vi "Scalar Bitpacked.vi"(8 "error in (no error)":errorcluster, 11 "Node Ptr":T1 format="%.0x") -> (0 "error out":errorcluster)   [LabVIEW 2015, in "FPGA Addon System Explorer.lvlib"]
uses:
  FPGA Addon System Explorer.lvlib
  <vilib>/NI Veristand/Custom Device API/Custom Device Item Ref.ctl
  Shared/FG Action.ctl
  <vilib>/NI Veristand/Custom Device API/Custom Device Channel.ctl
  <vilib>/NI Veristand/Custom Device API/Custom Device Channel Type.ctl
  Shared/Constants.vi
  <vilib>/NI Veristand/Custom Device API/Get Item Property (U32).vi
  <vilib>/NI Veristand/Custom Device API/NI VeriStand - Set Item Property.vi
  <vilib>/NI Veristand/Custom Device API/Set Item Property (U32).vi
  <vilib>/NI Veristand/Custom Device API/Get Item Property (String).vi
  <vilib>/NI Veristand/Custom Device API/Get Item Property (Variant).vi
  <vilib>/NI Veristand/Custom Device API/Set Item Property (Variant).vi
  <vilib>/NI Veristand/Custom Device Tools/Custom Device Utility Library/NI VeriStand - Search for All Items by GUID.vi
  <vilib>/NI VeriStand/Custom Device API/Custom Device API.lvlib
  Shared/FPGA Addon Shared.lvlib
  <vilib>/NI VeriStand/Custom Device Tools/Custom Device Utility Library/Custom Device Utility Library.lvlib
panel:
  out "Original Name":string
  in  "SHDocVw.IWebBrowser":refnum<k7>(container)
  in  "Reset":bool
  in  "Apply":bool
  in  "Number of Channels":u8
  in  "Header 2":cluster{"Section Name":string}={"Section Name"="Custom Device Item Settings"}
  in  "Header":cluster{"Section Name":string}={"Section Name"="Custom Device Item Settings"}
  in  "Description":string
  in  "Name":string
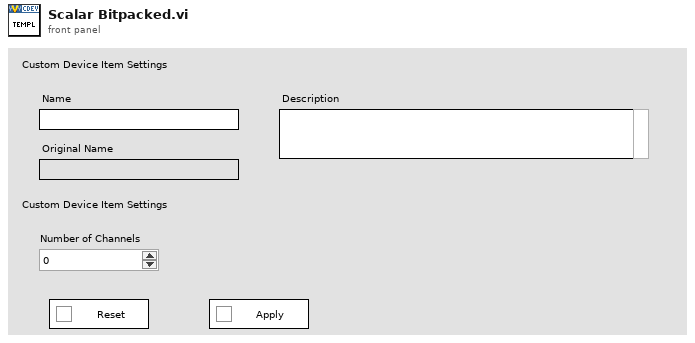
[diagram p1: front panel]
types:
  T1 = typedef "Custom Device API.lvlib/Custom Device Item Ref.ctl" = u64
  T2 = typedef "FPGA Addon Shared.lvlib/FG Action.ctl" = enum8{"GET", "SET"}
  T3 = typedef "FPGA Addon Shared.lvlib/Scalar Settings.ctl" = cluster{"Number of Channels":u8}
  T4 = typedef "FPGA Addon Shared.lvlib/Register Information.ctl" = cluster{"Name":string, "Data Type":T5, "Default Value":variant}
  T5 = typedef "FPGA Addon Shared.lvlib/Data Type.ctl" = enum8{"<Null>", "I8", "I16", "I32", "I64", "U8", "U16", "U32", "U64", "SGL", "Boolean", "Analog PWM In Settings", "Analog PWM In", "Digital PWM In Settings", "Digital PWM In", "Digital PWM Out", "Sine Out", "FXP+/-24.5", "FXP+/-16.5", "FXP+/-32.8", "FXP+/-64.32", "FXP+/-16.7", "FXP+/-20.5", "FXP+/-27.5", "FXP+/-32.16", "Digital Static In", "Digital Static Out", "Digital Static In Settings", "Digital WSS Out"}
  T6 = typedef "Custom Device API.lvlib/Custom Device Item Info.ctl" = cluster{"Name":string, "Is Channel":bool, "GUID":string, "Is Waveform":bool}
  T7 = typedef "Custom Device API.lvlib/Custom Device Channel.ctl" = cluster{"Type":T8, "Units":string, "Default Value":dbl, "Faultable":bool, "Scalable":bool}
  T8 = typedef "Custom Device API.lvlib/Custom Device Channel Type.ctl" = enum16{"Input", "Output"}
  T9 = typedef "Custom Device API.lvlib/Custom Device Commands.ctl" = enum16{"Default", "Item renamed", "Shutdown", "Dynamic button pressed"}
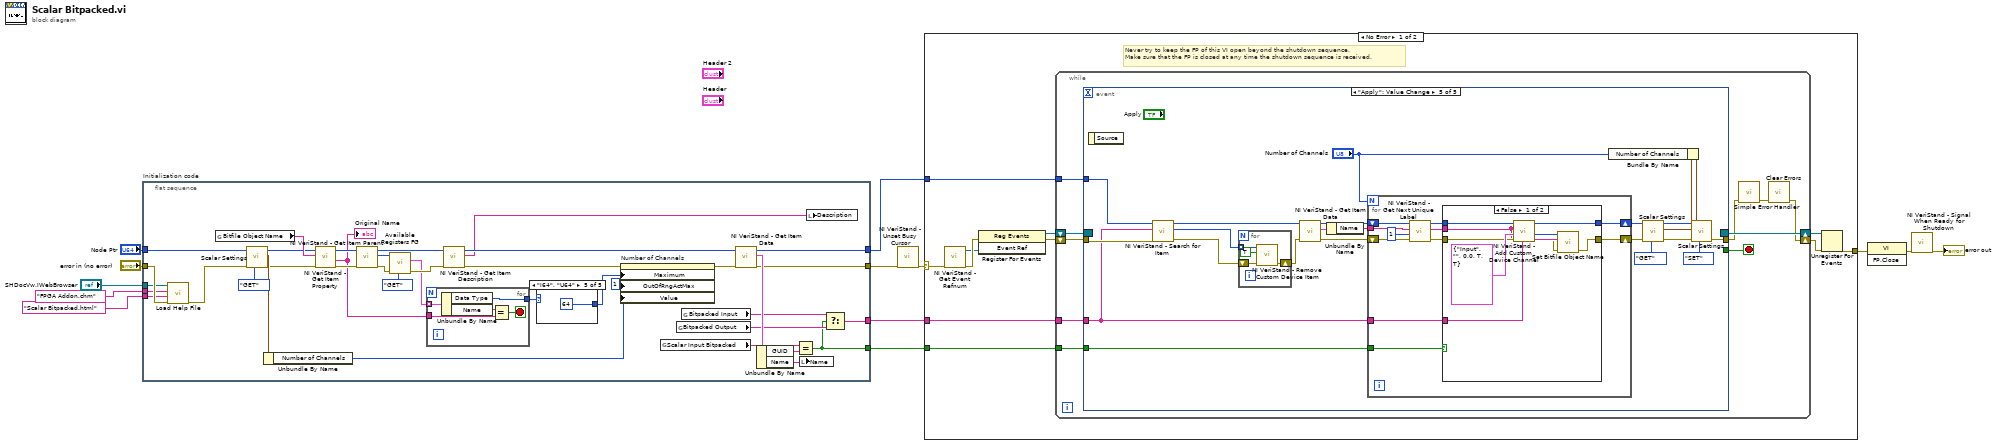
[diagram p0: block diagram]
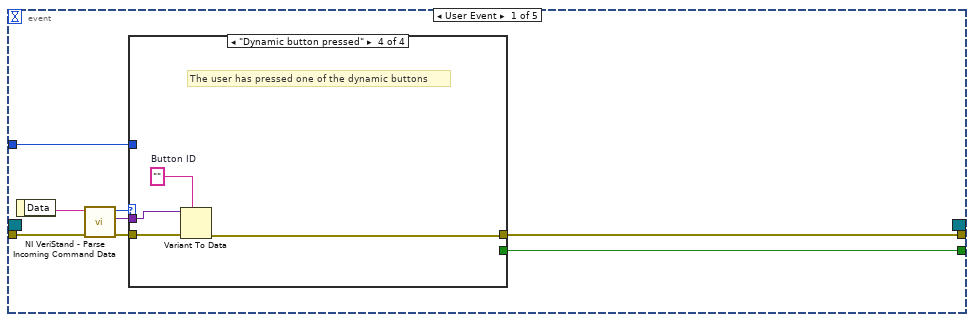
[diagram p2: hidden frame]
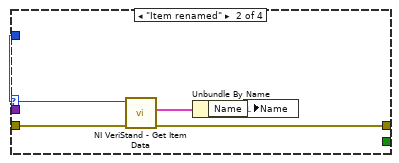
[diagram p4: hidden frame]
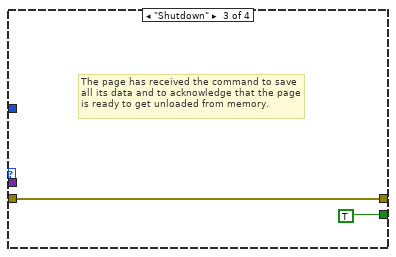
[diagram p5: hidden frame]
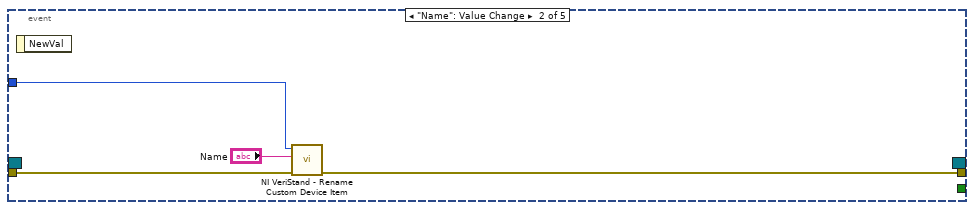
[diagram p6: hidden frame]
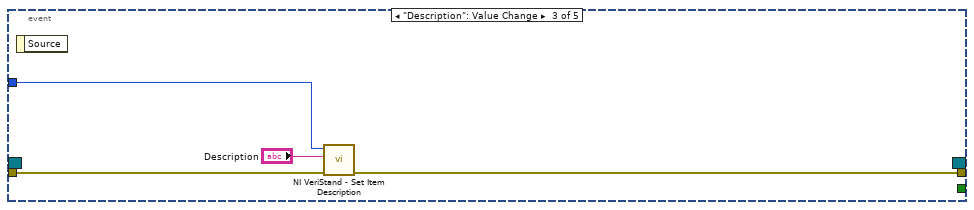
[diagram p7: hidden frame]
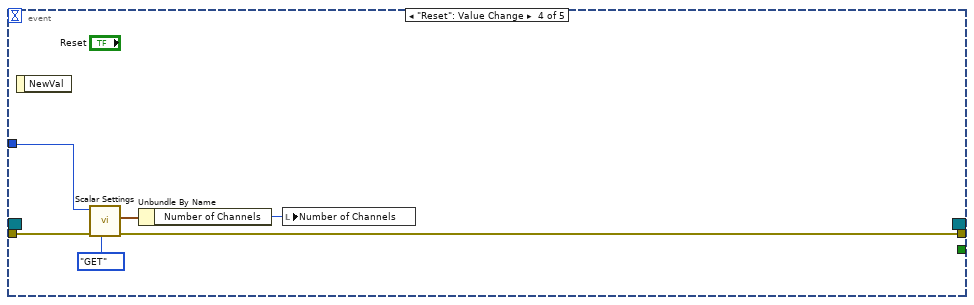
[diagram p8: hidden frame]
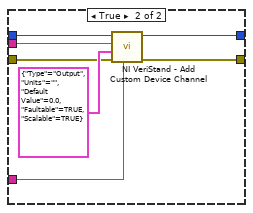
[diagram p9: hidden frame]
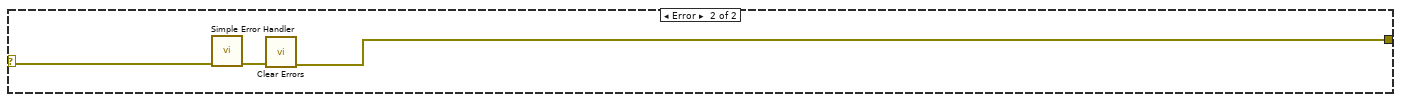
[diagram p10: hidden frame]
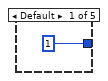
[diagram p11: hidden frame]
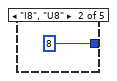
[diagram p12: hidden frame]
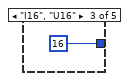
[diagram p13: hidden frame]
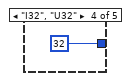
[diagram p14: hidden frame]
diagram:
  n1 = flat-sequence "Initialization code" {
    tunnel: "error in (no error)" -> [w19]
    tunnel: "Node Ptr" -> [w27]
    tunnel: [w47] -> w10
    tunnel: [w48] -> w8
    tunnel: [w43] -> w5
    tunnel: [w42] -> w4
    tunnel: "SHDocVw.IWebBrowser" -> [w17]
    tunnel: "FPGA Addon.chm" ("Main CHM File") -> [w16]
    tunnel: "Scalar Bitpacked.html" ("HTML File") -> [w15]
    frame #0 {
      n2 = call "Load Help File.vi"("error in (no error)"=w19, "HTML File"=w15, "Main CHM File"=w16, "SHDocVw.IWebBrowser2"=w17) -> ("error out"=w18:errorcluster)  [unwired: 7 in]
      n3 = global read "Constants.vi" "Bitfile Object Name"() -> (w32:string)
      n4 = call "Scalar Settings.vi"("Action"=FG_Action."GET", "error in (no error)"=w18, "Item Ref"=w27) -> ("error out"=w26:errorcluster, "Scalar Settings"=w39:T3, "Item Ref out"=w25:T1)  [unwired: 6 in]
      n5 = Unbundle By Name(w39) -> ("Number of Channels"=w30:u8)
      n6 = call-poly <vilib>:"NI VeriStand - Get Item Property.vi"("error in (no error)"=w26, "Property Name"=w32, "Item Ref in"=w25) -> ("error out"=w23:errorcluster, "Value"=w14:string, "Item Ref out"=w24:T1)  [unwired: 5 in, 1 out]
      "Original Name" <- w14
      n7 = call <vilib>:"NI VeriStand - Get Item Parent.vi"("error in (no error)"=w23, "Item Ref in"=w24) -> ("error out"=w36:errorcluster, "Parent Ref"=w37:T1, "Item Ref out"=w38:T1)  [unwired: 6 in, 1 out]
      n8 = call "Available Registers FG.vi"("Action"=FG_Action."GET", "error in (no error)"=w36, "Item Ref"=w37) -> ("error out"=w35:errorcluster, "Available Registers"=w33:T4[])  [unwired: 6 in, 1 out]
      n9 = for {
        tunnel: w33 -> [w61] mode=indexing
        tunnel: w14 -> [w59]
        tunnel: [w57] -> w29
        stop <- w58 stop-if-true
        n10 = Unbundle By Name(w61) -> ("Data Type"=w57:T5, "Name"=w60:string)
        n11 = Equal?(x=w60, y=w59) -> (x = y?=w58:bool)
      }
      n12 = call <vilib>:"NI VeriStand - Get Item Description.vi"("error in (no error)"=w35, "Item Ref in"=w38) -> ("error out"=w22:errorcluster, "Description"=w50:string, "Item Ref out"=w51:T1)  [unwired: 7 out]
      n13 = case shown="\"I64\", \"U64\"" w29 {
        tunnel: [1 8 16 32 64] -> w28
        frame Default {
        }
        frame "I8", "U8" {
        }
        frame "I16", "U16" {
        }
        frame "I32", "U32" {
        }
        frame "I64", "U64" {
        }
      }
      n14 = property on="Number of Channels" class="DigNum (strict)"(error in=w22, "Maximum"=w28, "OutOfRngActMax"=u8 1 ("Response to Value Outside Limits:Maximum"), "Value"=w30) -> (error out=w21:errorcluster)  [unwired: 1 in, 1 out]
      n15 = global read "Constants.vi" "Scalar Input Bitpacked"() -> (w46:string)
      n16 = global read "Constants.vi" "Bitpacked Output"() -> (w45:string)
      n17 = global read "Constants.vi" "Bitpacked Input"() -> (w44:string)
      n18 = call <vilib>:"NI VeriStand - Get Item Data.vi"("error in (no error)"=w21, "Item Ref in"=w51) -> ("error out"=w47:errorcluster, "Item Info"=w49:T6, "Item Ref out"=w48:T1)  [unwired: 7 out]
      n19 = Unbundle By Name(w49) -> ("GUID"=w41:string, "Name"=w20:string)
      n20 = Equal?(x=w46, y=w41) -> (x = y?=w43:bool)
      n21 = local write "Name"(w20) -> ()
      n22 = local write "Description"(w50) -> ()
      n23 = Select(t=w44, s=w43, f=w45) -> (s? t:f=w42:string)
    }
  }
  n24 = call <vilib>:"NI VeriStand - Unset Busy Cursor.vi"("error in (no error)"=w10) -> ("error out"=w9:errorcluster)  [unwired: 10 out]
  n25 = case shown="No Error" w9 {
    selector: w9 -> [w64 w172]
    tunnel: [w69 w170] -> w13
    tunnel: w8 -> [w65 _]
    tunnel: w5 -> [w63 _]
    tunnel: w4 -> [w62 _]
    frame No Error {
      # "Never try to keep the FP of this VI open beyond the shutdown sequence.\nMake sure that the FP is closed at any time the shutdown sequence is received."
      n26 = call <vilib>:"NI VeriStand - Get Event Refnum.vi"("error in (no error)"=w64) -> ("error out"=w72:errorcluster, "Event Ref"=w68:refnum<user-event>)  [unwired: 9 out]
      n27 = register-events(error in=w72, w68) -> (reference out=w66:refnum<event-registration>, error out=w67:errorcluster)  [unwired: 1 in]
      n28 = while {
        tunnel: w65 -> [w78]
        shift-right: [w75] -> w70
        shift-left: w67 -> [w81]
        shift-right: [w82] -> w71
        shift-left: w66 -> [w80]
        tunnel: w63 -> [w74]
        tunnel: w62 -> [w73]
        stop <- w79 stop-if-true
        n29 = event shown="[4] \"Apply\": Value Change" {
          selector: w80 -> [_ _ _ _ _]
          dyn-events: [_ _ _ _ _] -> w82
          timeout: _ -> [_ _ _ _ _]
          tunnel: w81 -> [w90 w106 w109 w116 w124]
          tunnel: [w86 _ _ _ _] -> w79
          tunnel: [w85 w105 w108 w112 w130] -> w77
          tunnel: w78 -> [w84 w104 w110 w114 w125]
          tunnel: w74 -> [_ _ _ _ w126]
          tunnel: w73 -> [_ _ _ _ w121]
          event User Event {
            n30 = event-data() -> ("Data"=w89:string)  [unwired: 1 out]
            n31 = call <vilib>:"NI VeriStand - Parse Incoming Command Data.vi"("error in (no error)"=w90, "Incoming data"=w89) -> ("error out"=w88:errorcluster, "Outgoing data"=w83:variant, "Action"=w87:T9)  [unwired: 7 out]
            n32 = case shown="\"Dynamic button pressed\"" w87 {
              tunnel: w88 -> [w91 w96 w97 w102]
              tunnel: [_ _ TRUE _] -> w86
              tunnel: [w91 w93 w97 w99] -> w85
              tunnel: w84 -> [_ w95 _ _]
              tunnel: w83 -> [_ _ _ w101]
              frame "Default", Default {
              }
              frame "Item renamed" {
                n33 = call <vilib>:"NI VeriStand - Get Item Data.vi"("error in (no error)"=w96, "Item Ref in"=w95) -> ("error out"=w93:errorcluster, "Item Info"=w94:T6)  [unwired: 8 out]
                n34 = Unbundle By Name(w94) -> ("Name"=w92:string)
                n35 = local write "Name"(w92) -> ()
              }
              frame "Shutdown" {
                # "The page has received the command to save all its data and to acknowledge that the page is ready to get unloaded from memory."
              }
              frame "Dynamic button pressed" {
                w100 = ""  # Button ID
                # "The user has pressed one of the dynamic buttons"
                n36 = Variant To Data(error in=w102, type=w100, Variant=w101) -> (error out=w99:errorcluster)  [unwired: 1 out]
              }
            }
          }
          event "Name": Value Change {
            n37 = event-data() -> ()  [unwired: 2 out]
            n38 = call <vilib>:"NI VeriStand - Rename Custom Device Item.vi"("error in (no error)"=w106, "New Name"="Name", "Item Ref in"=w104) -> ("error out"=w105:errorcluster)  [unwired: 1 in, 7 out]
          }
          event "Description": Value Change {
            n39 = event-data() -> ()  [unwired: 2 out]
            n40 = call <vilib>:"NI VeriStand - Set Item Description.vi"("error in (no error)"=w109, "Description"="Description", "Item Ref in"=w110) -> ("error out"=w108:errorcluster)  [unwired: 8 out]
          }
          event "Reset": Value Change {
            n41 = event-data() -> ()  [unwired: 2 out]
            n42 = call "Scalar Settings.vi"("Action"=FG_Action."GET", "error in (no error)"=w116, "Item Ref"=w114) -> ("error out"=w112:errorcluster, "Scalar Settings"=w113:T3)  [unwired: 6 in, 1 out]
            n43 = Unbundle By Name(w113) -> ("Number of Channels"=w111:u8)
            n44 = local write "Number of Channels"(w111) -> ()
          }
          event "Apply": Value Change {
            n45 = event-data() -> ()  [unwired: 2 out]
            n46 = call-poly <vilib>:"NI VeriStand - Search for Item.vi"("error in"=w124, "Item GUID"=w121, "Section Ref in"=w125) -> ("error out"=w122:errorcluster, "Item Refs"=w120:T1[], "Section Ref out"=w123:T1)  [unwired: 5 in, 1 out]
            n47 = for {
              shift-right: [w141] -> w137
              shift-left: w122 -> [w142]
              tunnel: w120 -> [w139] mode=indexing
              n48 = call <vilib>:"NI VeriStand - Remove Custom Device Item.vi"("error in (no error)"=w142, "Force Delete (F)"=TRUE, "Item Ref in"=w139) -> ("error out"=w141:errorcluster)  [unwired: 7 in, 1 out]
            }
            n49 = call <vilib>:"NI VeriStand - Get Item Data.vi"("error in (no error)"=w137, "Item Ref in"=w123) -> ("error out"=w119:errorcluster, "Item Info"=w136:T6, "Item Ref out"=w117:T1)  [unwired: 7 out]
            n50 = Unbundle By Name(w136) -> ("Name"=w118:string)
            n51 = for {
              N: "Number of Channels" -> [_]
              tunnel: w118 -> [w147]
              shift-right: [w153] -> w135
              shift-left: w119 -> [w149]
              shift-right: [w145] -> w134
              shift-left: w117 -> [w148]
              tunnel: w121 -> [w144]
              tunnel: w126 -> [w143]
              n52 = call <vilib>:"NI VeriStand - Get Next Unique Label.vi"("error in (no error)"=w149, "Start Value (1)"=1, "Label"=w147, "Parent Ref in"=w148) -> ("error out"=w152:errorcluster, "Label out"=w150:string, "Parent Ref dup"=w151:T1)  [unwired: 4 in, 1 out]
              n53 = case shown="False" w143 {
                tunnel: [w154 w165] -> w153
                tunnel: w152 -> [w160 w166]
                tunnel: w151 -> [w161 w168]
                tunnel: w150 -> [w156 w167]
                tunnel: [w159 w164] -> w145
                tunnel: w144 -> [w158 w163]
                frame False {
                  n54 = call <vilib>:"NI VeriStand - Add Custom Device Channel.vi"("GUID (Default Channel)"=w158, "error in (no error)"=w160, "Channel"=T7 {"Type"=enum."Input", "Units"="", "Default Value"=0.0, "Faultable"=TRUE, "Scalable"=TRUE}, "Channel Name"=w156, "Parent Ref in"=w161) -> ("error out"=w155:errorcluster, "Channel Ref"=w157:T1, "Parent Ref out"=w159:T1)  [unwired: 3 in, 1 out]
                  n55 = call "Set Bitfile Object Name.vi"("error in (no error)"=w155, "Name"=w156, "Channel Ref"=w157) -> ("error out"=w154:errorcluster)  [unwired: 8 in]
                }
                frame True {
                  n56 = call <vilib>:"NI VeriStand - Add Custom Device Channel.vi"("GUID (Default Channel)"=w163, "error in (no error)"=w166, "Channel"=T7 {"Type"=enum."Output", "Units"="", "Default Value"=0.0, "Faultable"=TRUE, "Scalable"=TRUE}, "Channel Name"=w167, "Parent Ref in"=w168) -> ("error out"=w165:errorcluster, "Parent Ref out"=w164:T1)  [unwired: 3 in, 2 out]
                }
              }
            }
            n57 = call "Scalar Settings.vi"("Action"=FG_Action."GET", "error in (no error)"=w135, "Item Ref"=w134) -> ("error out"=w131:errorcluster, "Scalar Settings"=w129:T3, "Item Ref out"=w132:T1)  [unwired: 6 in]
            n58 = Bundle By Name(cluster=w129, "Number of Channels"="Number of Channels") -> (w128:T3)
            n59 = call "Scalar Settings.vi"("Action"=FG_Action."SET", "error in (no error)"=w131, "Scalar Settings"=w128, "Item Ref"=w132) -> ("error out"=w130:errorcluster)  [unwired: 5 in, 2 out]
          }
        }
        n60 = call <vilib>:"Simple Error Handler.vi"("error in (no error)"=w77) -> ("error out"=w76:errorcluster)  [unwired: 1 in, 7 out]
        n61 = call <vilib>:"Clear Errors.vi"("error in (no error)"=w76) -> ("error out"=w75:errorcluster)  [unwired: 1 in, 5 out]
      }
      n62 = Unregister For Events(event registration refnum=w71, error in=w70) -> (error out=w69:errorcluster)
    }
    frame Error {
      n63 = call <vilib>:"Simple Error Handler.vi"("error in (no error)"=w172) -> ("error out"=w171:errorcluster)  [unwired: 1 in, 7 out]
      n64 = call <vilib>:"Clear Errors.vi"("error in (no error)"=w171) -> ("error out"=w170:errorcluster)  [unwired: 1 in, 5 out]
    }
  }
  n65 = invoke class="VI" method="FP.Close"(error in=w13) -> (error out=w12:errorcluster)  [unwired: 2 in, 2 out]
  n66 = call <vilib>:"NI VeriStand - Signal When Ready for Shutdown.vi"("error in (no error)"=w12) -> ("error out"=→"error out":errorcluster)  [unwired: 10 out]
